vi "Initialize Remote Terminals.vi"(8 "error in":errorcluster, 9 "next available buffer id":u16, 10 "remote terminals":T1[](array[typedef]), 11 "module handle":u32) -> (0 "error out":errorcluster, 1 "next available buffer id out":u16, 2 "rt address to buffer id map":T3, 3 "module handle out":u32)   [LabVIEW 2020, in "AIM MIL-STD-1553 Engine.lvlib" / "Implementation.lvlib" / "Shared Resources.lvclass"]
uses:
  Shared Resources.lvclass
  RT Subaddress to Buffer ID Map.ctl
  Shared/Direction.ctl
  Custom Device/Remote Terminal Configuration.ctl
  <instrlib>/_AIM MIL-STD-1553/AIM Controls/1553 Select Direction.ctl
  Hardware API/AIM MIL-STD-1553 Hardware API.lvlib
  Custom Device/Custom Device.lvlib
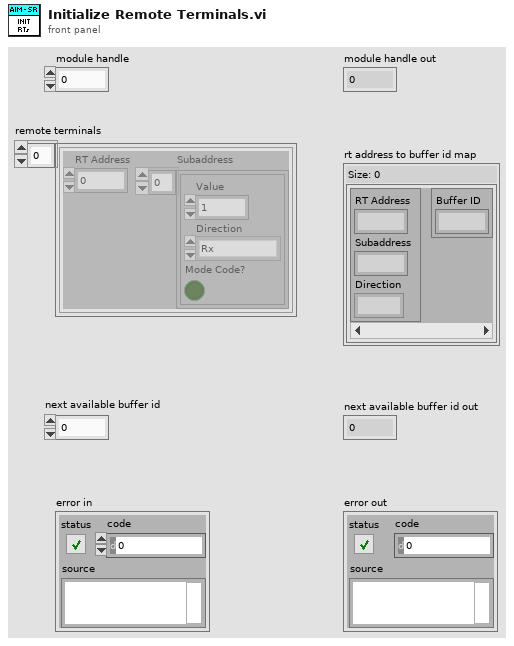
[diagram p1: front panel]
types:
  T1 = typedef "AIM MIL-STD-1553 Engine.lvlib/Custom Device.lvlib/Remote Terminal Configuration.ctl" = cluster{"RT Address":u8, "Subaddress":cluster{"Value":u8, "Direction":T2, "Mode Code?":bool}[]}
  T2 = typedef "Direction.ctl" = enum16{"Rx", "Tx"}
  T3 = typedef "AIM MIL-STD-1553 Engine.lvlib/Implementation.lvlib/Shared Resources.lvclass/RT Subaddress to Buffer ID Map.ctl" = map{cluster{"RT Address":u8, "Subaddress":u8, "Direction":T2}, cluster{"Buffer ID":u16}}
  T4 = typedef "1553 Select Direction.ctl" = enum16{"receive", "transmit"}
  T5 = cluster{"Value":u8, "Direction":T2, "Mode Code?":bool}[]
  T6 = cluster{"RT Address":u8, "mode code\nsubaddress":i32, "Direction":T2}
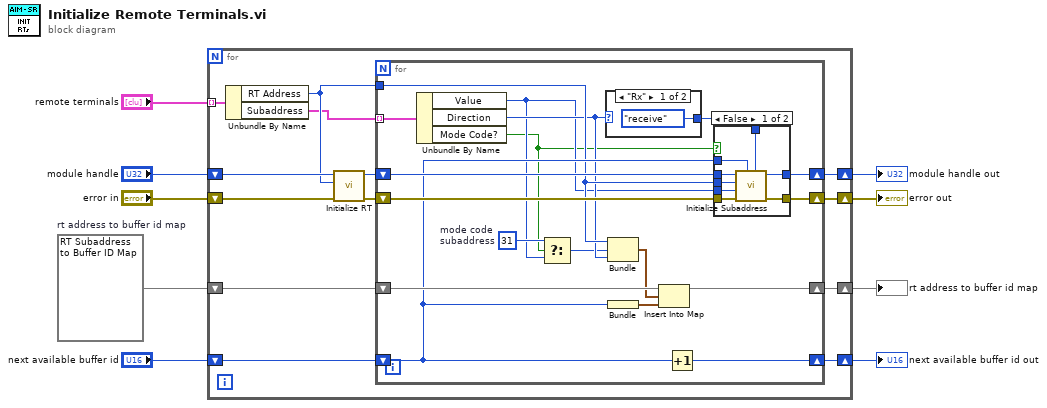
[diagram p0: block diagram]
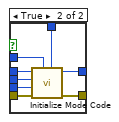
[diagram p2: hidden frame]
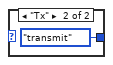
[diagram p3: hidden frame]
diagram:
  w7 = T3 {}  # rt address to buffer id map
  n1 = for {
    shift-right: [w19] -> w5
    shift-left: "module handle" -> [w22]
    shift-right: [w18] -> w6
    shift-left: "error in" -> [w21]
    tunnel: "remote terminals" -> [w16] mode=indexing
    shift-right: [w12] -> w9
    shift-left: "next available buffer id" -> [w13]
    shift-right: [w10] -> w4
    shift-left: w7 -> [w11]
    n2 = Unbundle By Name(w16) -> ("RT Address"=w15:u8, "Subaddress"=w14:T5)
    n3 = call "Initialize RT.vi"("error in"=w21, "rt address"=w15, "module handle"=w22) -> ("error out"=w17:errorcluster, "module handle out"=w20:u32)  [unwired: 7 in]
    n4 = for {
      shift-right: [w39] -> w19
      shift-left: w20 -> [w40]
      shift-right: [w37] -> w18
      shift-left: w17 -> [w38]
      tunnel: w15 -> [w30]
      tunnel: w14 -> [w36] mode=indexing
      shift-right: [w34] -> w12
      shift-left: w13 -> [w31]
      shift-right: [w32] -> w10
      shift-left: w11 -> [w33]
      w26 = 31  # mode code subaddress
      n5 = Unbundle By Name(w36) -> ("Value"=w25:u8, "Direction"=w28:T2, "Mode Code?"=w23:bool)
      n6 = Select(t=w26, s=w23, f=w25) -> (s? t:f=w24:i32)
      n7 = case shown="\"Rx\"" w28 {
        tunnel: [1553_Select_Direction."receive" ("Direction (receive)") 1553_Select_Direction."transmit" ("Direction (receive)")] -> w35
        frame "Rx" {
        }
        frame "Tx" {
        }
      }
      n8 = Bundle("RT Address"=w30, "mode code\nsubaddress"=w24, "Direction"=w28) -> (w29:T6)  [unwired: 1 in]
      n9 = Bundle("next available buffer id"=w31) -> (w27:cluster{"next available buffer id":u16})  [unwired: 1 in]
      n10 = Insert Into Map(map in=w33, key=w29, value=w27) -> (map out=w32:T3)  [unwired: 2 out]
      n11 = Increment(x=w31) -> (x+1=w34:u16)
      n12 = case shown="False" w23 {
        tunnel: w40 -> [w48 w54]
        tunnel: [w47 w49] -> w39
        tunnel: w38 -> [w46 w56]
        tunnel: [w45 w55] -> w37
        tunnel: w35 -> [w44 w50]
        tunnel: w31 -> [w43 w51]
        tunnel: w30 -> [w42 w53]
        tunnel: w25 -> [w41 w52]
        frame False {
          n13 = call "Initialize Subaddress.vi"("direction (receive)"=w44, "buffer header and buffer id"=w43, "error in"=w46, "subaddress"=w41, "remote terminal address"=w42, "module handle"=w48) -> ("error out"=w45:errorcluster, "module handle out"=w47:u32)  [unwired: 4 in]
        }
        frame True {
          n14 = call "Initialize Mode Code.vi"("direction (receive)"=w50, "buffer header and buffer id"=w51, "error in"=w56, "mode code"=w52, "remote terminal address"=w53, "module handle"=w54) -> ("error out"=w55:errorcluster, "module handle out"=w49:u32)  [unwired: 4 in]
        }
      }
    }
  }
  "next available buffer id out" <- w9
  "error out" <- w6
  "module handle out" <- w5
  "rt address to buffer id map" <- w4
